vi "rs3 Set All Advanced4.vi"(0 "Set Color Corr":bool=TRUE, 1 "Depth Presets":T2(ring), 2 "Color Presets":T1(ring), 7 "error in (no error)":errorcluster, 8 "device in":u64=370866768, 10 "ST_CensusEnable":cluster{"uDiameter":u32, "vDiameter":u32}={"uDiameter"=9, "vDiameter"=9}, 12 "ST_AE_Control":cluster{"meanIntensitySetpoint":u32}={"meanIntensitySetpoint"=400}, 16 "Depth Table":T3={"depthUnits, um"=1000, "depthClampMin"=0, "depthClampMax"=65535, "disparityMultiplier"=0, "disparityShift"=0}, 17 "ST RAU vector":T9={"minWest"=1, "minEast"=1, "minWEsum"=1, "minNorth"=1, "minSouth"=1, "minNSSum"=1, "uStrink"=1, "vShrink"=1}, 19 "ST Color Control":T8, 20 "depth control":T4={"plusIncrement"=10, "MinusDecrement"=10, "deepSeaMedianThreshold"=528, "scoreThreshA"=10, "scoreThreshB"=1023, "textureDifferenceThreshold"=0, "textureCountThreshold"=0, "deepSeaSecondPeakThreshold"=27, "deepSeaNeighborThreshold"=20, "IrAgreeThreshold"=70}, 21 "STColorCorrection":T11={"colorCorrection 1"=0.54785156, "colorCorrection 2"=0.32910156, "colorCorrection 3"=0.8222656, "colorCorrection 4"=0.109375, "colorCorrection 5"=-0.40527344, "colorCorrection 6"=-1.5253906, "colorCorrection 7"=0.95703125, "colorCorrection 8"=0.89160156, "colorCorrection 9"=0.7675781, "colorCorrection 10"=-0.4794922, "colorCorrection 11"=0.047851562, "colorCorrection 12"=-0.2705078}, 22 "HDAD":T12={"lambdaCensus"=26.0, "lambdaAD"=2100.0, "ignoreSAD"=0}, 23 "ST RSM":T10={"rsmBypass"=0, "diffThresh"=7.0, "sloRauDiffThresh"=3.0, "removeThresh"=33}, 24 "ST SLO Penalty":T5={"sloK1Penalty"=44, "sloK2Penalty"=502, "sloK1PenaltyMod1"=23, "sloK2PenaltyMod1"=237, "sloK1PenaltyMod2"=219, "sloK2PenaltyMod2"=113}, 25 "ST SLO Threshold":T6={"SLOdiffThresholdRed"=300, "SLODiffThresholdGreen"=300, "SLODiffThresholdBlue"=300}, 26 "ST Rau Threshold":T7={"rauDiffThresholdRed"=600, "rauDiffThresholdGreen"=600, "rauDiffThresholdBlue"=600}) -> (14 "Set advanced error":string, 18 "Dev out":u64=370866768, 27 "error out":errorcluster)   [LabVIEW 2017, in "libRealSense3.lvlib"]
doc: "The RealSense D4xx cameras are based on a stereo algorithm that has been accelerated as a fixed-function inside an ASIC. There are many parameters that affect the calculation of the depth. The basic task is to solve the correspondance problem - i.e. figure out which patches in the left image match up to those in the right image by doing a search along an epipolar line (x-axis). The x-axis difference for each object point is known as the disparity. \n\nIn general depth can be estimated for most points in the scene, but some points will have a very low confidence because 1. they are may be occluded (not seen by both imagers), or 2. have very little texture on them which will lead to an ambiquity (ex. when looking at a completely uniform white wall it, there are no best correspondances).\n\nThis VI allows you to set the many parameters that affect the algorith, as well as the color reproduction. \nNote that the color correction matrix will NOT have any effect on the depth calculations."
uses:
  <vilib>/addons/RealSense/libRealSense3.lvlib
panel:
  # "RS3 Set All Advanced 4"
  # "(C) 2017 Intel Corp.,  AGJ"
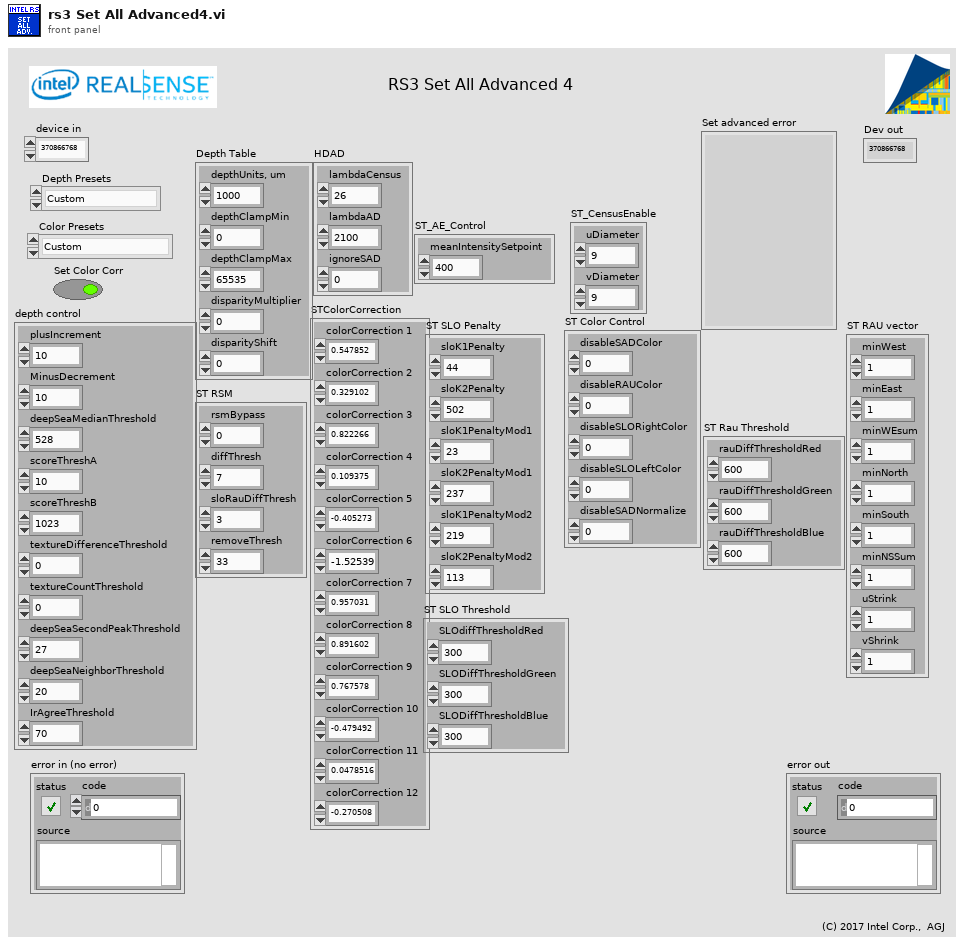
[diagram p1: front panel]
types:
  T1 = enum16{"Custom", "RS400 (DS5p)", "RS400 (DS5p) 2", "RS400 (DS5p) 3", "RS400 (DS5p) 4", "RS400 (DS5p) 5", "RS410 (DS5a)", "RS410 (DS5a) 2", "DS410 (DS5a) 3", "DS410 (DS5a) 4", "DS410+IR", "DS5LR", "DS5LR-2", "DS5LR no pattern", "RS410 Remove IR", "RS410 Remove IR 2", "DS5micro", "D435"}
  T2 = enum16{"Custom", "Original", "New Depth 1", "New Depth 2", "Depth Active 1", "Active 3D Scan", "Active Short A", "Active Short C", "Face", "Face2", "Best Box", "High Density", "Medium Density", "High Accuracy", "Hand", "Short Range", "Flat wall", "Load .JSON", "Load .JSON2"}
  T3 = cluster{"depthUnits, um":u32, "depthClampMin":u32, "depthClampMax":u32, "disparityMultiplier":u32, "disparityShift":u32}
  T4 = cluster{"plusIncrement":u32, "MinusDecrement":u32, "deepSeaMedianThreshold":u32, "scoreThreshA":u32, "scoreThreshB":u32, "textureDifferenceThreshold":u32, "textureCountThreshold":u32, "deepSeaSecondPeakThreshold":u32, "deepSeaNeighborThreshold":u32, "IrAgreeThreshold":u32}
  T5 = cluster{"sloK1Penalty":u32, "sloK2Penalty":u32, "sloK1PenaltyMod1":u32, "sloK2PenaltyMod1":u32, "sloK1PenaltyMod2":u32, "sloK2PenaltyMod2":u32}
  T6 = cluster{"SLOdiffThresholdRed":u32, "SLODiffThresholdGreen":u32, "SLODiffThresholdBlue":u32}
  T7 = cluster{"rauDiffThresholdRed":u32, "rauDiffThresholdGreen":u32, "rauDiffThresholdBlue":u32}
  T8 = cluster{"disableSADColor":u32, "disableRAUColor":u32, "disableSLORightColor":u32, "disableSLOLeftColor":u32, "disableSADNormalize":u32}
  T9 = cluster{"minWest":u32, "minEast":u32, "minWEsum":u32, "minNorth":u32, "minSouth":u32, "minNSSum":u32, "uStrink":u32, "vShrink":u32}
  T10 = cluster{"rsmBypass":u32, "diffThresh":sgl, "sloRauDiffThresh":sgl, "removeThresh":u32}
  T11 = cluster{"colorCorrection 1":sgl, "colorCorrection 2":sgl, "colorCorrection 3":sgl, "colorCorrection 4":sgl, "colorCorrection 5":sgl, "colorCorrection 6":sgl, "colorCorrection 7":sgl, "colorCorrection 8":sgl, "colorCorrection 9":sgl, "colorCorrection 10":sgl, "colorCorrection 11":sgl, "colorCorrection 12":sgl}
  T12 = cluster{"lambdaCensus":sgl, "lambdaAD":sgl, "ignoreSAD":u32}
  T13 = cluster{"rsmBypass (56)":u32, "diffThresh (57)":sgl, "sloRauDiffThresh(58)":sgl, "removeThresh(59)":u32}
  T14 = cluster{"depth control":cluster{"plusIncrement":u32, "MinusDecrement":u32, "deepSeaMedianThreshold":u32, "scoreThreshA":u32, "scoreThreshB":u32, "textureDifferenceThreshold":u32, "textureCountThreshold":u32, "deepSeaSecondPeakThreshold":u32, "deepSeaNeighborThreshold":u32, "IrAgreeThreshold":u32}, "STColorCorrection output":cluster{"colorCorrection 1":sgl, "colorCorrection 2":sgl, "colorCorrection 3":sgl, "colorCorrection 4":sgl, "colorCorrection 5":sgl, "colorCorrection 6":sgl, "colorCorrection 7":sgl, "colorCorrection 8":sgl, "colorCorrection 9":sgl, "colorCorrection 10":sgl, "colorCorrection 11":sgl, "colorCorrection 12":sgl}, "HDAD":cluster{"lambdaCensus":sgl, "lambdaAD":sgl, "ignoreSAD":u32}, "ST RSM":cluster{"rsmBypass":u32, "diffThresh":sgl, "sloRauDiffThresh":sgl, "removeThresh":u32}, "ST SLO Penalty":cluster{"sloK1Penalty":u32, "sloK2Penalty":u32, "sloK1PenaltyMod1":u32, "sloK2PenaltyMod1":u32, "sloK1PenaltyMod2":u32, "sloK2PenaltyMod2":u32}, "ST SLO Threshold":cluster{"SLOdiffThresholdRed":u32, "SLODiffThresholdGreen":u32, "SLODiffThresholdBlue":u32}, "ST Rau Threshold":cluster{"rauDiffThresholdRed":u32, "rauDiffThresholdGreen":u32, "rauDiffThresholdBlue":u32}, "ST Color Control":cluster{"disableSADColor":u32, "disableRAUColor":u32, "disableSLORightColor":u32, "disableSLOLeftColor":u32, "disableSADNormalize":u32}, "ST RAU vector":cluster{"minWest":u32, "minEast":u32, "minWEsum":u32, "minNorth":u32, "minSouth":u32, "minNSSum":u32, "uStrink":u32, "vShrink":u32}, "Depth Table":cluster{"depthUnits, um":u32, "depthClampMin":u32, "depthClampMax":u32, "disparityMultiplier":u32, "disparityShift":u32}, "ST_AE_Control":cluster{"meanIntensitySetpoint":u32}, "ST_CensusEnable":cluster{"uDiameter":u32, "vDiameter":u32}}
  T15 = cluster{"depthUnits, um":u32, "depthClampMin":u32, "depthClampMax":u32, "disparityMultiplier":u32, "disparityShift(0-127)":u32}
  T16 = cluster{"minWest (60)":u32, "minEast (61)":u32, "minWEsum (62)":u32, "minNorth (63)":u32, "minSouth (64)":u32, "minNSSum(65)":u32, "uStrink (66)":u32, "vShrink (67)":u32}
  T17 = cluster{"rauDiffThreshRed(73)":u32, "rauDiffThreshGreen(74)":u32, "rauDiffThreshBlue(75)":u32}
  T18 = cluster{"sloK1Penalty (79)":u32, "sloK2Penalty (80)":u32, "sloK1PenaltyMod1(81)":u32, "sloK2PenaltyMod1(82)":u32, "sloK1PenaltyMod2(83)":u32, "sloK2PenaltyMod2(84)":u32}
  T19 = cluster{"SLOdiffThreshRed(76)":u32, "SLODiffThreshGreen(77)":u32, "SLODiffThreshBlue(78)":u32}
  T20 = cluster{"disableSADColor(68)":u32, "disableRAUColor(69)":u32, "disableSLORightColor(70)":u32, "disableSLOLeftColor(71)":u32, "disableSADNormalize(72)":u32}
  T21 = cluster{"plusIncrement (47)":u32, "MinusDecrement (46)":u32, "deepSeaMedianThreshold (48)":u32, "scoreThreshA(49)":u32, "scoreThreshB (50)":u32, "textureDifferenceThreshold (52)":u32, "textureCountThreshold (51)":u32, "deepSea2ndPeakThresh.(53)":u32, "deepSeaNeighborThresh.(54)":u32, "LRAgreeThreshold (55)":u32}
  T22 = cluster{"plusIncrement (47)":u32, "MinusDecrement (46)":u32, "deepSeaMedianThreshold (48)":u32, "scoreThreshA(49)":u32, "scoreThreshB (50)":u32, "textureDifferenceThreshold (52)":u32, "textureCountThreshold (51)":u32, "deepSea2ndPeakThresh.(53)":u32, "deepSeaNeighborThresh.(54)":u32, "IrAgreeThreshold (55)":u32}
  T23 = cluster{"DS5p- 1":sgl, "colorCorrection 2":sgl, "colorCorrection 3":sgl, "colorCorrection 4":sgl, "colorCorrection 5":sgl, "colorCorrection 6":sgl, "colorCorrection 7":sgl, "colorCorrection 8":sgl, "colorCorrection 9":sgl, "colorCorrection 10":sgl, "colorCorrection 11":sgl, "colorCorrection 12":sgl}
  T24 = cluster{"Color 0":dbl, "Color 1":dbl, "Color 2":dbl, "Color 3":dbl, "Color 4":dbl, "Color 5":dbl, "Color 6":dbl, "Color 7":dbl, "Color 8":dbl, "Color 9":dbl, "Color 10":dbl, "Color 11":dbl}
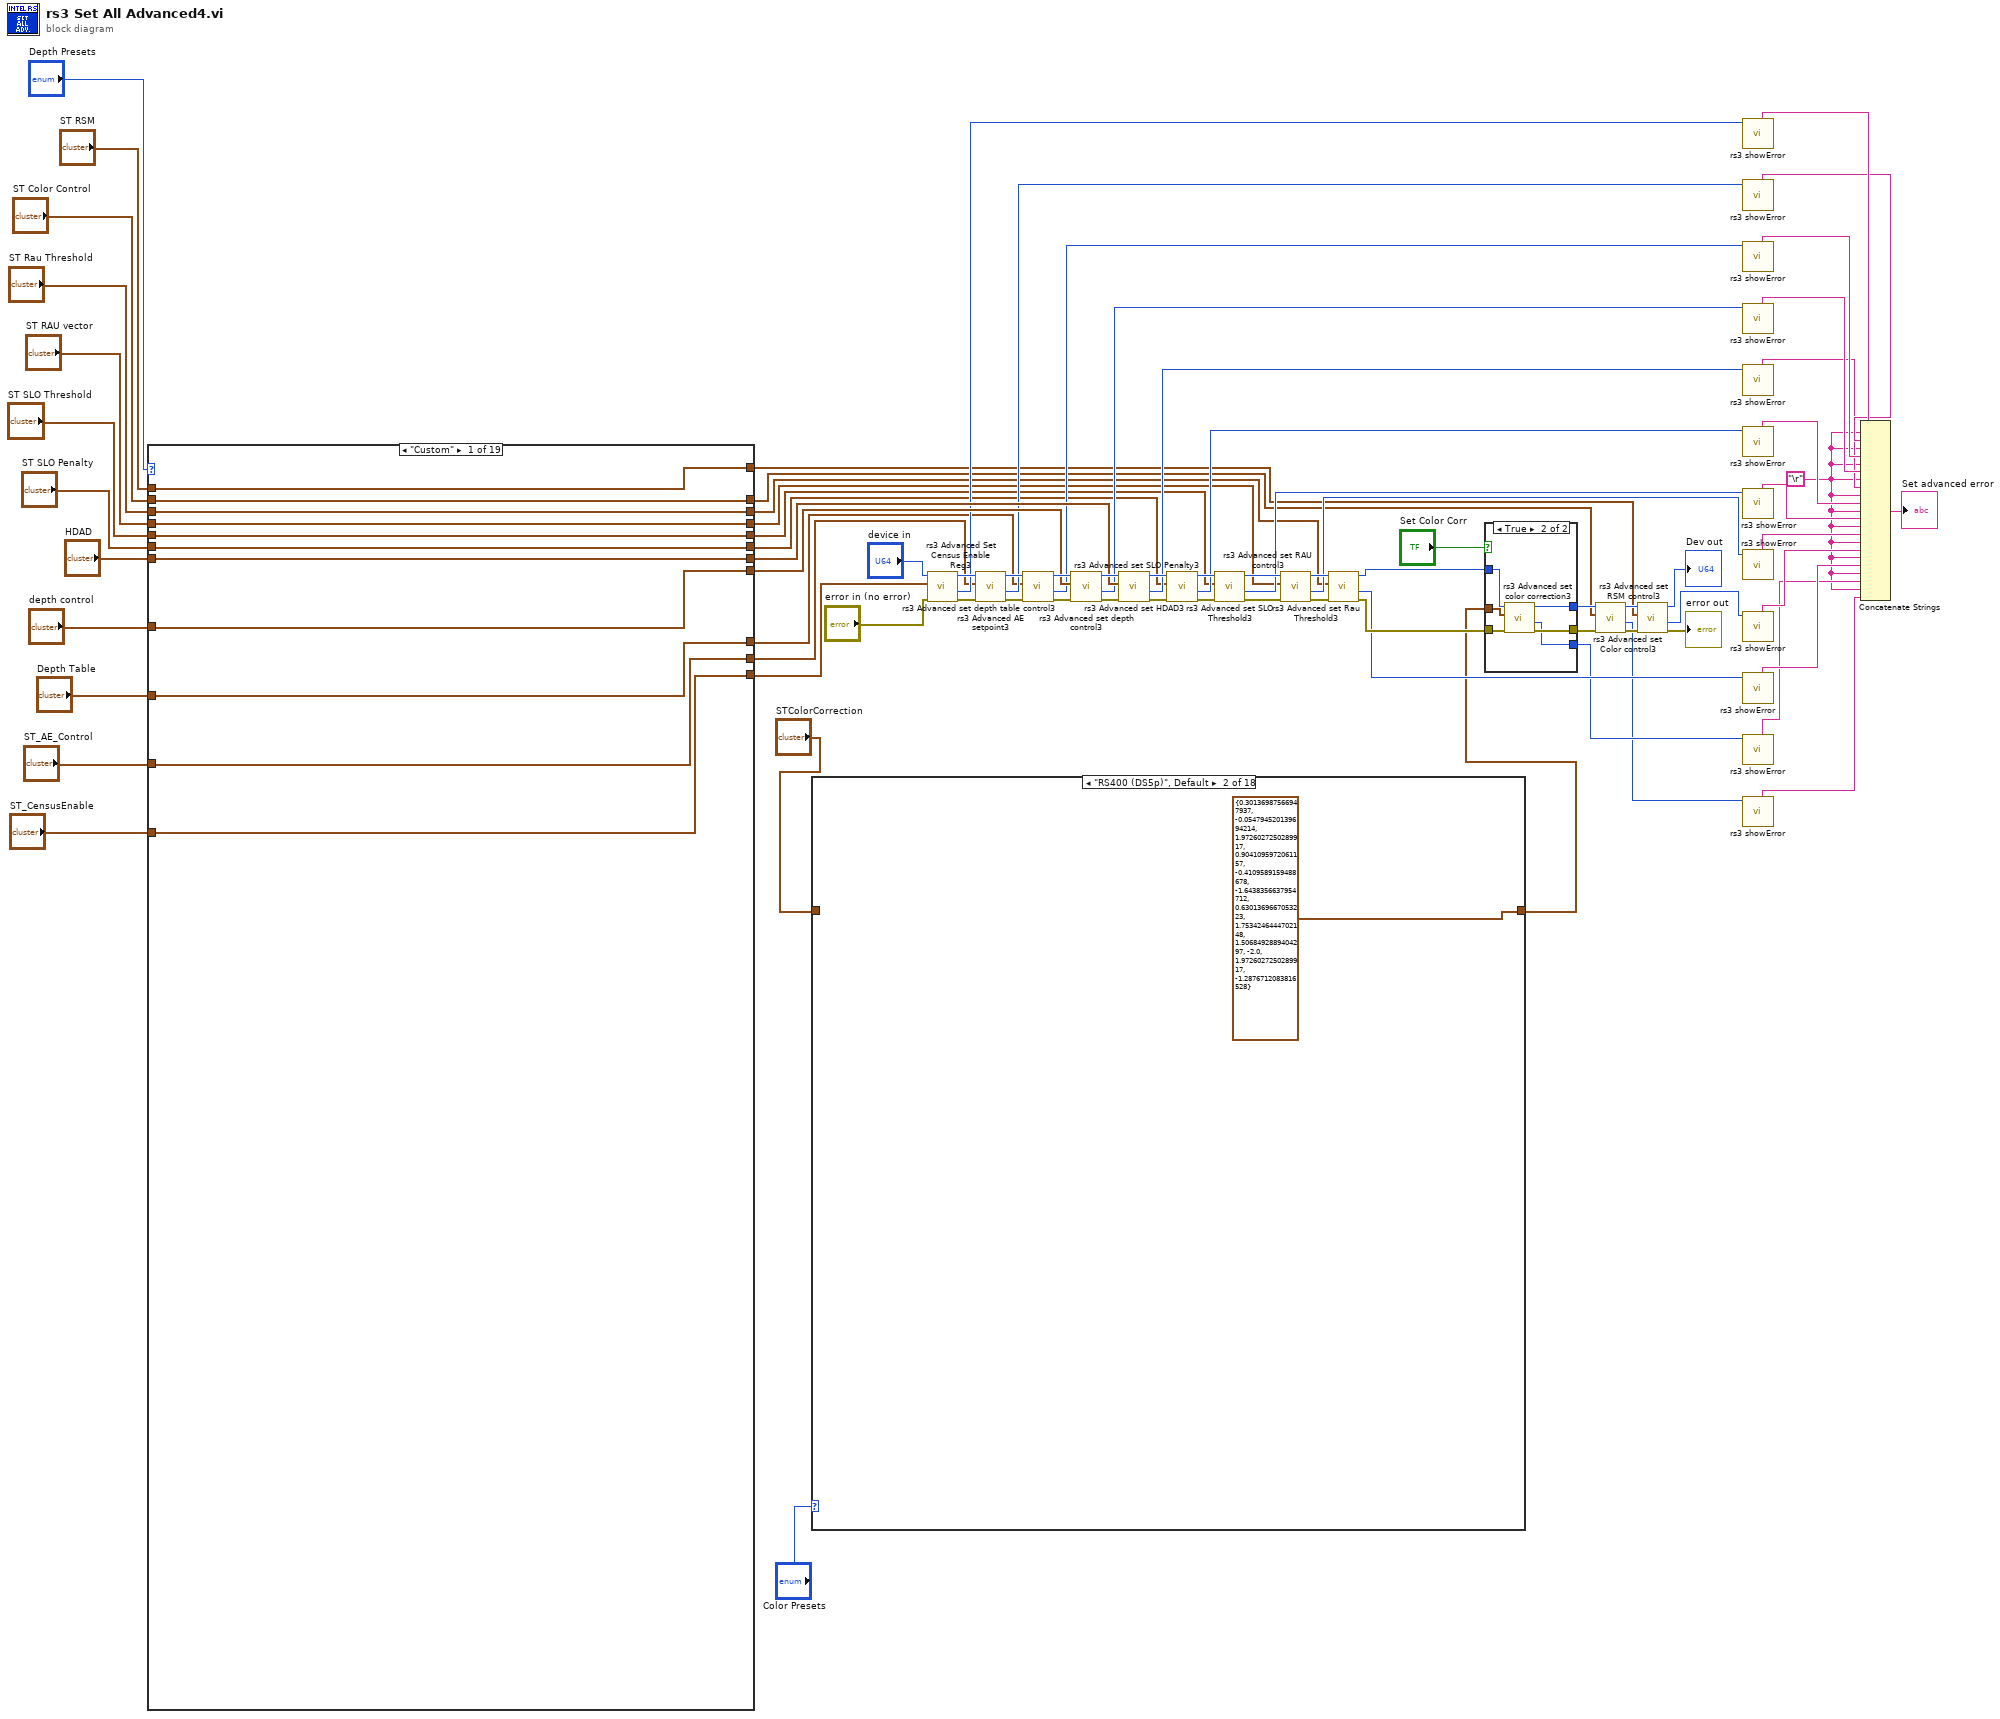
[diagram p0: block diagram]
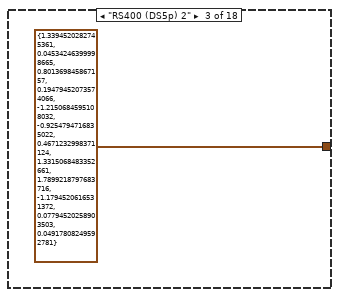
[diagram p3: hidden frame]
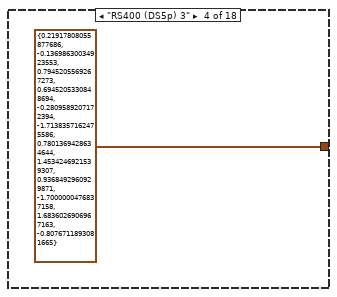
[diagram p4: hidden frame]
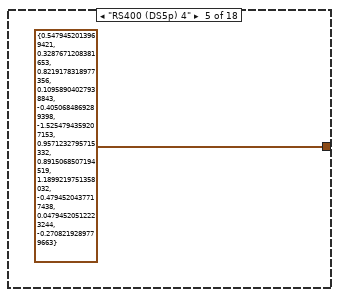
[diagram p5: hidden frame]
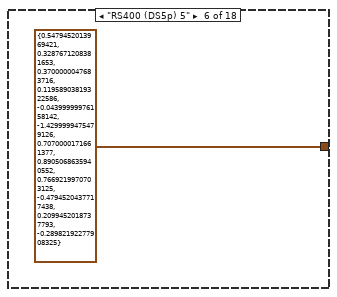
[diagram p6: hidden frame]
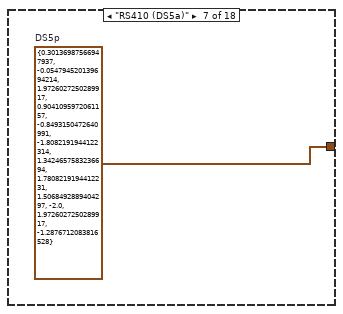
[diagram p7: hidden frame]
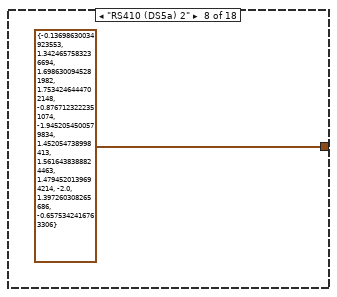
[diagram p8: hidden frame]
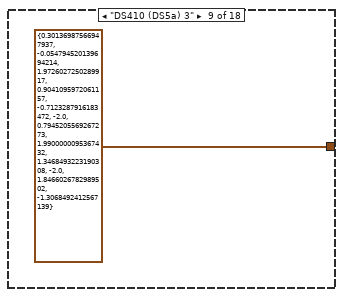
[diagram p9: hidden frame]
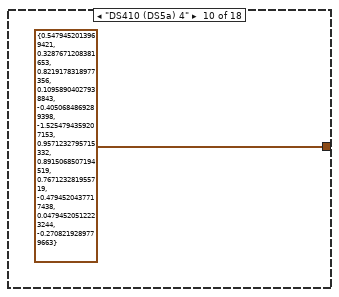
[diagram p10: hidden frame]
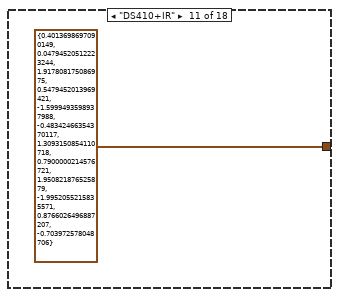
[diagram p11: hidden frame]
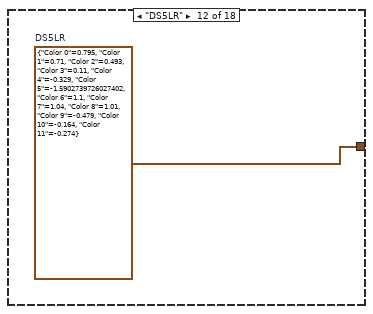
[diagram p12: hidden frame]
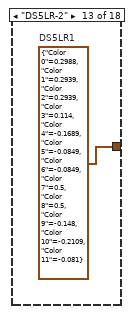
[diagram p13: hidden frame]
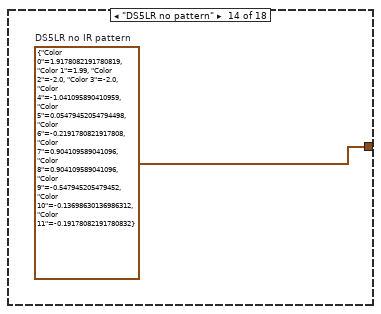
[diagram p14: hidden frame]
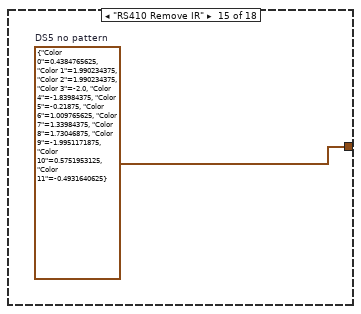
[diagram p15: hidden frame]
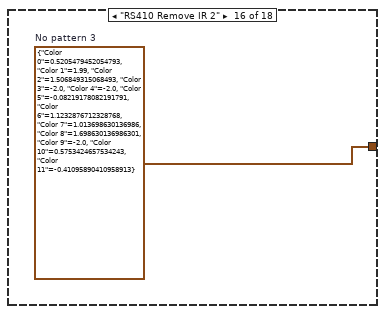
[diagram p16: hidden frame]
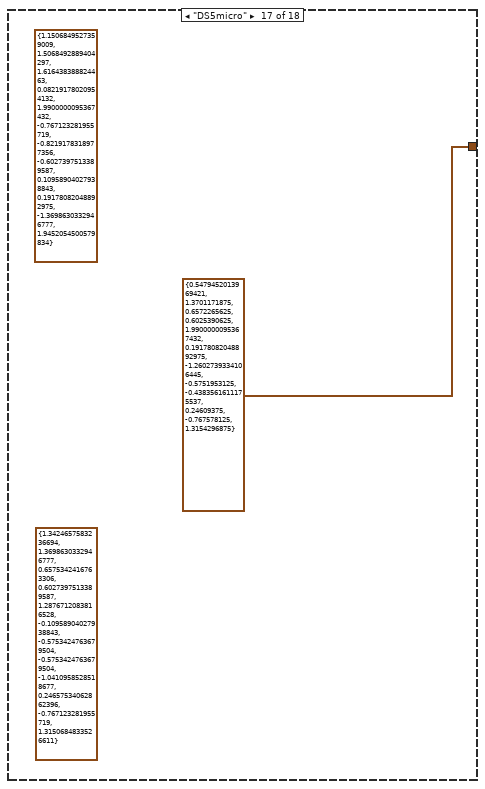
[diagram p17: hidden frame]
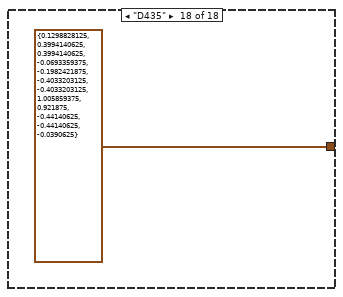
[diagram p18: hidden frame]
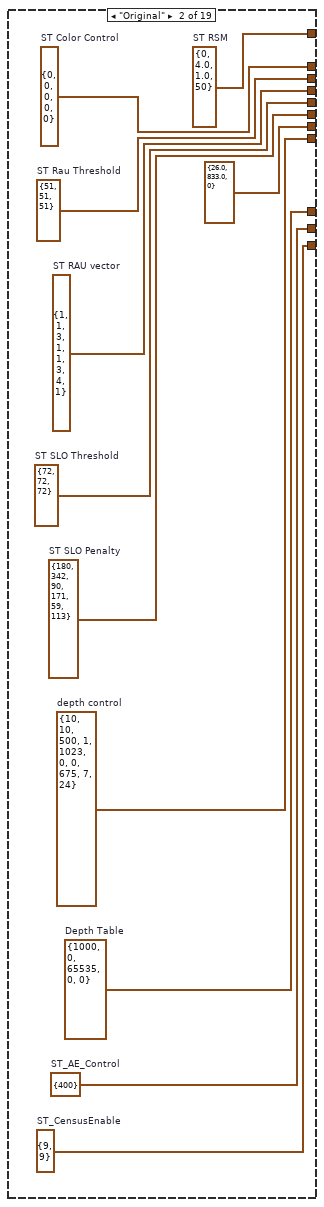
[diagram p19: hidden frame]
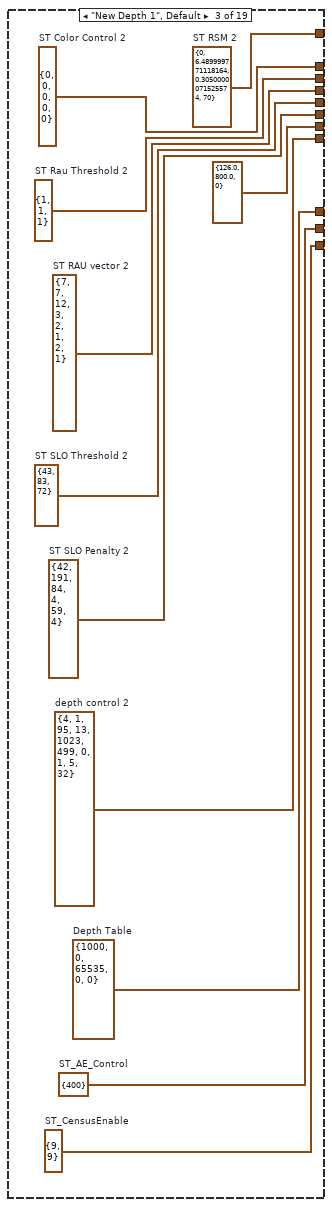
[diagram p20: hidden frame]
diagram:
  w23 = "\r"
  n1 = case shown="\"Custom\"" "Depth Presets" {
    tunnel: [w90 w100 w112 w123 w134 w138 w149 w160 w176 w186 w197 w204 w217 w229 w241 w253 w265 w280 w294] -> w50
    tunnel: [w84 w99 w111 w122 w133 T13 {"rsmBypass (56)"=0, "diffThresh (57)"=1.0367311, "sloRauDiffThresh(58)"=151.0, "removeThresh(59)"=1} ("ST RSM 2") w156 w167 w178 w183 w194 w209 w222 w234 w246 w258 w270 w282 w296] -> w12
    tunnel: [w85 w94 w110 w121 w132 w145 w155 w166 w177 w184 w195 w211 w224 w236 w248 w260 w272 w279 w293] -> w14
    tunnel: [w86 w95 w109 w120 w131 w144 w154 w165 w174 w185 w196 w207 w220 w232 w244 w256 w268 w283 w297] -> w15
    tunnel: [w83 w98 w108 w119 w130 w143 w153 w164 w173 w187 w198 w203 w216 w228 w240 w252 w264 w286 w300] -> w10
    tunnel: [w87 w97 w107 w118 w129 w142 w152 w163 w171 w188 w199 w202 w215 w227 w239 w251 w263 w285 w299] -> w17
    tunnel: [w88 w96 w106 w117 w128 w141 w151 w162 w175 w189 w200 w201 w214 w226 w238 w250 w262 w284 w298] -> w20
    tunnel: [w89 T12 {"lambdaCensus"=26.0, "lambdaAD"=833.0, "ignoreSAD"=0} ("HDAD 2") T12 {"lambdaCensus"=126.0, "lambdaAD"=800.0, "ignoreSAD"=0} ("HDAD 2") T12 {"lambdaCensus"=200.0, "lambdaAD"=1900.0, "ignoreSAD"=0} ("HDAD 2") T12 {"lambdaCensus"=216.0, "lambdaAD"=1400.0, "ignoreSAD"=0} ("HDAD 2") T12 {"lambdaCensus"=26.0, "lambdaAD"=833.0, "ignoreSAD"=0} ("HDAD 2") T12 {"lambdaCensus"=100.0, "lambdaAD"=1600.0, "ignoreSAD"=0} ("HDAD 2") w161 w172 T12 {"lambdaCensus"=26.0, "lambdaAD"=2100.0, "ignoreSAD"=0} ("HDAD*") T12 {"lambdaCensus"=15.0, "lambdaAD"=618.0, "ignoreSAD"=0} ("HDAD*") w210 w223 w235 w247 w259 w271 w281 w295] -> w48
    tunnel: [w81 w91 w102 w113 w124 w135 w146 w158 w168 w179 w190 w205 w218 w230 w242 w254 w266 w273 w289] -> w6
    tunnel: [w82 w92 w103 w114 w125 w136 w147 w157 w169 w180 w191 w206 w219 w231 w243 w255 w267 w274 w288] -> w8
    tunnel: [w80 w93 w104 w115 w126 w137 w148 w159 w170 w181 w192 w208 w221 w233 w245 w257 w269 w275 w287] -> w4
    tunnel: "depth control" -> [w90 _ _ _ _ _ _ _ _ _ _ _ _ _ _ _ _ _ _]
    tunnel: "HDAD" -> [w89 _ _ _ _ _ _ _ _ _ _ _ _ _ _ _ _ _ _]
    tunnel: "ST SLO Penalty" -> [w88 _ _ _ _ _ _ _ _ _ _ _ _ _ _ _ _ _ _]
    tunnel: "ST SLO Threshold" -> [w87 _ _ _ _ _ _ _ _ _ _ _ _ _ _ _ _ _ _]
    tunnel: "ST RAU vector" -> [w85 _ _ _ _ _ _ _ _ _ _ _ _ _ _ _ _ _ _]
    tunnel: "ST Rau Threshold" -> [w86 _ _ _ _ _ _ _ _ _ _ _ _ _ _ _ _ _ _]
    tunnel: "ST RSM" -> [w84 _ _ _ _ _ _ _ _ _ _ _ _ _ _ _ _ _ _]
    tunnel: "ST Color Control" -> [w83 _ _ _ _ _ _ _ _ _ _ _ _ _ _ _ _ _ _]
    tunnel: "ST_CensusEnable" -> [w82 _ _ _ _ _ _ _ _ _ _ _ _ _ _ _ _ _ _]
    tunnel: "ST_AE_Control" -> [w81 _ _ _ _ _ _ _ _ _ _ _ _ _ _ _ _ _ _]
    tunnel: "Depth Table" -> [w80 _ _ _ _ _ _ _ _ _ _ _ _ _ _ _ _ _ _]
    frame "Custom" {
    }
    frame "Original" {
      w92 = cluster{"uDiameter":u32, "vDiameter":u32} {"uDiameter"=9, "vDiameter"=9}  # ST_CensusEnable
      w93 = T15 {"depthUnits, um"=1000, "depthClampMin"=0, "depthClampMax"=65535, "disparityMultiplier"=0, "disparityShift(0-127)"=0}  # Depth Table
      w91 = cluster{"meanIntensitySetpoint":u32} {"meanIntensitySetpoint"=400}  # ST_AE_Control
      w94 = T16 {"minWest (60)"=1, "minEast (61)"=1, "minWEsum (62)"=3, "minNorth (63)"=1, "minSouth (64)"=1, "minNSSum(65)"=3, "uStrink (66)"=4, "vShrink (67)"=1}  # ST RAU vector
      w95 = T17 {"rauDiffThreshRed(73)"=51, "rauDiffThreshGreen(74)"=51, "rauDiffThreshBlue(75)"=51}  # ST Rau Threshold
      w96 = T18 {"sloK1Penalty (79)"=180, "sloK2Penalty (80)"=342, "sloK1PenaltyMod1(81)"=90, "sloK2PenaltyMod1(82)"=171, "sloK1PenaltyMod2(83)"=59, "sloK2PenaltyMod2(84)"=113}  # ST SLO Penalty
      w97 = T19 {"SLOdiffThreshRed(76)"=72, "SLODiffThreshGreen(77)"=72, "SLODiffThreshBlue(78)"=72}  # ST SLO Threshold
      w98 = T20 {"disableSADColor(68)"=0, "disableRAUColor(69)"=0, "disableSLORightColor(70)"=0, "disableSLOLeftColor(71)"=0, "disableSADNormalize(72)"=0}  # ST Color Control
      w99 = T13 {"rsmBypass (56)"=0, "diffThresh (57)"=4.0, "sloRauDiffThresh(58)"=1.0, "removeThresh(59)"=50}  # ST RSM
      w100 = T21 {"plusIncrement (47)"=10, "MinusDecrement (46)"=10, "deepSeaMedianThreshold (48)"=500, "scoreThreshA(49)"=1, "scoreThreshB (50)"=1023, "textureDifferenceThreshold (52)"=0, "textureCountThreshold (51)"=0, "deepSea2ndPeakThresh.(53)"=675, "deepSeaNeighborThresh.(54)"=7, "LRAgreeThreshold (55)"=24}  # depth control
    }
    frame "New Depth 1", Default {
      w103 = cluster{"uDiameter":u32, "vDiameter":u32} {"uDiameter"=9, "vDiameter"=9}  # ST_CensusEnable
      w104 = T15 {"depthUnits, um"=1000, "depthClampMin"=0, "depthClampMax"=65535, "disparityMultiplier"=0, "disparityShift(0-127)"=0}  # Depth Table
      w102 = cluster{"meanIntensitySetpoint":u32} {"meanIntensitySetpoint"=400}  # ST_AE_Control
      w106 = T18 {"sloK1Penalty (79)"=42, "sloK2Penalty (80)"=191, "sloK1PenaltyMod1(81)"=84, "sloK2PenaltyMod1(82)"=4, "sloK1PenaltyMod2(83)"=59, "sloK2PenaltyMod2(84)"=4}  # ST SLO Penalty 2
      w107 = T19 {"SLOdiffThreshRed(76)"=43, "SLODiffThreshGreen(77)"=83, "SLODiffThreshBlue(78)"=72}  # ST SLO Threshold 2
      w108 = T20 {"disableSADColor(68)"=0, "disableRAUColor(69)"=0, "disableSLORightColor(70)"=0, "disableSLOLeftColor(71)"=0, "disableSADNormalize(72)"=0}  # ST Color Control 2
      w109 = T17 {"rauDiffThreshRed(73)"=1, "rauDiffThreshGreen(74)"=1, "rauDiffThreshBlue(75)"=1}  # ST Rau Threshold 2
      w110 = T16 {"minWest (60)"=7, "minEast (61)"=7, "minWEsum (62)"=12, "minNorth (63)"=3, "minSouth (64)"=2, "minNSSum(65)"=1, "uStrink (66)"=2, "vShrink (67)"=1}  # ST RAU vector 2
      w111 = T13 {"rsmBypass (56)"=0, "diffThresh (57)"=6.49, "sloRauDiffThresh(58)"=0.305, "removeThresh(59)"=70}  # ST RSM 2
      w112 = T22 {"plusIncrement (47)"=4, "MinusDecrement (46)"=1, "deepSeaMedianThreshold (48)"=95, "scoreThreshA(49)"=13, "scoreThreshB (50)"=1023, "textureDifferenceThreshold (52)"=499, "textureCountThreshold (51)"=0, "deepSea2ndPeakThresh.(53)"=1, "deepSeaNeighborThresh.(54)"=5, "IrAgreeThreshold (55)"=32}  # depth control 2
    }
    frame "New Depth 2" {
      w114 = cluster{"uDiameter":u32, "vDiameter":u32} {"uDiameter"=9, "vDiameter"=9}  # ST_CensusEnable
      w115 = T15 {"depthUnits, um"=1000, "depthClampMin"=0, "depthClampMax"=65535, "disparityMultiplier"=0, "disparityShift(0-127)"=0}  # Depth Table
      w113 = cluster{"meanIntensitySetpoint":u32} {"meanIntensitySetpoint"=400}  # ST_AE_Control
      w117 = T18 {"sloK1Penalty (79)"=42, "sloK2Penalty (80)"=191, "sloK1PenaltyMod1(81)"=84, "sloK2PenaltyMod1(82)"=4, "sloK1PenaltyMod2(83)"=59, "sloK2PenaltyMod2(84)"=4}  # ST SLO Penalty 2
      w118 = T19 {"SLOdiffThreshRed(76)"=100, "SLODiffThreshGreen(77)"=100, "SLODiffThreshBlue(78)"=100}  # ST SLO Threshold 2
      w119 = T20 {"disableSADColor(68)"=0, "disableRAUColor(69)"=0, "disableSLORightColor(70)"=0, "disableSLOLeftColor(71)"=0, "disableSADNormalize(72)"=0}  # ST Color Control 2
      w120 = T17 {"rauDiffThreshRed(73)"=50, "rauDiffThreshGreen(74)"=50, "rauDiffThreshBlue(75)"=50}  # ST Rau Threshold 2
      w121 = T16 {"minWest (60)"=1, "minEast (61)"=1, "minWEsum (62)"=9, "minNorth (63)"=3, "minSouth (64)"=2, "minNSSum(65)"=1, "uStrink (66)"=2, "vShrink (67)"=1}  # ST RAU vector 2
      w122 = T13 {"rsmBypass (56)"=0, "diffThresh (57)"=6.49, "sloRauDiffThresh(58)"=0.305, "removeThresh(59)"=50}  # ST RSM 2
      w123 = T22 {"plusIncrement (47)"=4, "MinusDecrement (46)"=1, "deepSeaMedianThreshold (48)"=95, "scoreThreshA(49)"=13, "scoreThreshB (50)"=1023, "textureDifferenceThreshold (52)"=499, "textureCountThreshold (51)"=0, "deepSea2ndPeakThresh.(53)"=1, "deepSeaNeighborThresh.(54)"=5, "IrAgreeThreshold (55)"=200}  # depth control 2
    }
    frame "Depth Active 1" {
      w125 = cluster{"uDiameter":u32, "vDiameter":u32} {"uDiameter"=9, "vDiameter"=9}  # ST_CensusEnable
      w126 = T15 {"depthUnits, um"=1000, "depthClampMin"=0, "depthClampMax"=65535, "disparityMultiplier"=0, "disparityShift(0-127)"=0}  # Depth Table
      w124 = cluster{"meanIntensitySetpoint":u32} {"meanIntensitySetpoint"=400}  # ST_AE_Control
      w128 = T18 {"sloK1Penalty (79)"=10, "sloK2Penalty (80)"=60, "sloK1PenaltyMod1(81)"=84, "sloK2PenaltyMod1(82)"=56, "sloK1PenaltyMod2(83)"=59, "sloK2PenaltyMod2(84)"=4}  # ST SLO Penalty 2
      w129 = T19 {"SLOdiffThreshRed(76)"=200, "SLODiffThreshGreen(77)"=200, "SLODiffThreshBlue(78)"=200}  # ST SLO Threshold 2
      w130 = T20 {"disableSADColor(68)"=0, "disableRAUColor(69)"=0, "disableSLORightColor(70)"=0, "disableSLOLeftColor(71)"=0, "disableSADNormalize(72)"=0}  # ST Color Control 2
      w131 = T17 {"rauDiffThreshRed(73)"=70, "rauDiffThreshGreen(74)"=70, "rauDiffThreshBlue(75)"=70}  # ST Rau Threshold 2
      w132 = T16 {"minWest (60)"=7, "minEast (61)"=7, "minWEsum (62)"=12, "minNorth (63)"=3, "minSouth (64)"=2, "minNSSum(65)"=1, "uStrink (66)"=2, "vShrink (67)"=1}  # ST RAU vector 2
      w133 = T13 {"rsmBypass (56)"=0, "diffThresh (57)"=6.49, "sloRauDiffThresh(58)"=0.305, "removeThresh(59)"=60}  # ST RSM 2
      w134 = T22 {"plusIncrement (47)"=4, "MinusDecrement (46)"=1, "deepSeaMedianThreshold (48)"=95, "scoreThreshA(49)"=13, "scoreThreshB (50)"=1023, "textureDifferenceThreshold (52)"=499, "textureCountThreshold (51)"=0, "deepSea2ndPeakThresh.(53)"=1, "deepSeaNeighborThresh.(54)"=5, "IrAgreeThreshold (55)"=82}  # depth control 2
    }
    frame "Active 3D Scan" {
      w136 = cluster{"uDiameter":u32, "vDiameter":u32} {"uDiameter"=9, "vDiameter"=9}  # ST_CensusEnable
      w137 = T15 {"depthUnits, um"=1000, "depthClampMin"=0, "depthClampMax"=65535, "disparityMultiplier"=0, "disparityShift(0-127)"=0}  # Depth Table
      w135 = cluster{"meanIntensitySetpoint":u32} {"meanIntensitySetpoint"=400}  # ST_AE_Control
      w138 = T22 {"plusIncrement (47)"=19, "MinusDecrement (46)"=4, "deepSeaMedianThreshold (48)"=554, "scoreThreshA(49)"=1, "scoreThreshB (50)"=632, "textureDifferenceThreshold (52)"=0, "textureCountThreshold (51)"=31, "deepSea2ndPeakThresh.(53)"=665, "deepSeaNeighborThresh.(54)"=126, "IrAgreeThreshold (55)"=11}  # depth control 2
      w141 = T18 {"sloK1Penalty (79)"=93, "sloK2Penalty (80)"=473, "sloK1PenaltyMod1(81)"=70, "sloK2PenaltyMod1(82)"=123, "sloK1PenaltyMod2(83)"=92, "sloK2PenaltyMod2(84)"=409}  # ST SLO Penalty 2
      w142 = T19 {"SLOdiffThreshRed(76)"=46, "SLODiffThreshGreen(77)"=442, "SLODiffThreshBlue(78)"=105}  # ST SLO Threshold 2
      w143 = T20 {"disableSADColor(68)"=0, "disableRAUColor(69)"=0, "disableSLORightColor(70)"=0, "disableSLOLeftColor(71)"=0, "disableSADNormalize(72)"=0}  # ST Color Control 2
      w144 = T17 {"rauDiffThreshRed(73)"=46, "rauDiffThreshGreen(74)"=442, "rauDiffThreshBlue(75)"=105}  # ST Rau Threshold 2
      w145 = T16 {"minWest (60)"=5, "minEast (61)"=7, "minWEsum (62)"=12, "minNorth (63)"=1, "minSouth (64)"=3, "minNSSum(65)"=7, "uStrink (66)"=4, "vShrink (67)"=1}  # ST RAU vector 2
    }
    frame "Active Short A" {
      w147 = cluster{"uDiameter":u32, "vDiameter":u32} {"uDiameter"=3, "vDiameter"=3}  # ST_CensusEnable
      w148 = T15 {"depthUnits, um"=200, "depthClampMin"=0, "depthClampMax"=65535, "disparityMultiplier"=0, "disparityShift(0-127)"=0}  # Depth Table
      w146 = cluster{"meanIntensitySetpoint":u32} {"meanIntensitySetpoint"=400}  # ST_AE_Control
      w149 = T22 {"plusIncrement (47)"=7, "MinusDecrement (46)"=1, "deepSeaMedianThreshold (48)"=140, "scoreThreshA(49)"=10, "scoreThreshB (50)"=1023, "textureDifferenceThreshold (52)"=499, "textureCountThreshold (51)"=0, "deepSea2ndPeakThresh.(53)"=1, "deepSeaNeighborThresh.(54)"=5, "IrAgreeThreshold (55)"=80}  # depth control 2
      w151 = T18 {"sloK1Penalty (79)"=5, "sloK2Penalty (80)"=30, "sloK1PenaltyMod1(81)"=11, "sloK2PenaltyMod1(82)"=50, "sloK1PenaltyMod2(83)"=56, "sloK2PenaltyMod2(84)"=15}  # ST SLO Penalty 2
      w152 = T19 {"SLOdiffThreshRed(76)"=200, "SLODiffThreshGreen(77)"=200, "SLODiffThreshBlue(78)"=200}  # ST SLO Threshold 2
      w153 = T20 {"disableSADColor(68)"=0, "disableRAUColor(69)"=0, "disableSLORightColor(70)"=0, "disableSLOLeftColor(71)"=0, "disableSADNormalize(72)"=0}  # ST Color Control 2
      w154 = T17 {"rauDiffThreshRed(73)"=200, "rauDiffThreshGreen(74)"=200, "rauDiffThreshBlue(75)"=200}  # ST Rau Threshold 2
      w155 = T16 {"minWest (60)"=3, "minEast (61)"=3, "minWEsum (62)"=13, "minNorth (63)"=1, "minSouth (64)"=1, "minNSSum(65)"=1, "uStrink (66)"=4, "vShrink (67)"=4}  # ST RAU vector 2
      w156 = T13 {"rsmBypass (56)"=0, "diffThresh (57)"=7.5, "sloRauDiffThresh(58)"=0.9, "removeThresh(59)"=72}  # ST RSM 2
    }
    frame "Active Short C" {
      w157 = cluster{"uDiameter":u32, "vDiameter":u32} {"uDiameter"=3, "vDiameter"=3}  # ST_CensusEnable
      w159 = T15 {"depthUnits, um"=200, "depthClampMin"=0, "depthClampMax"=65535, "disparityMultiplier"=0, "disparityShift(0-127)"=0}  # Depth Table
      w158 = cluster{"meanIntensitySetpoint":u32} {"meanIntensitySetpoint"=400}  # ST_AE_Control
      w160 = T22 {"plusIncrement (47)"=10, "MinusDecrement (46)"=10, "deepSeaMedianThreshold (48)"=415, "scoreThreshA(49)"=1, "scoreThreshB (50)"=1023, "textureDifferenceThreshold (52)"=0, "textureCountThreshold (51)"=14, "deepSea2ndPeakThresh.(53)"=56, "deepSeaNeighborThresh.(54)"=108, "IrAgreeThreshold (55)"=8}  # depth control 2
      w161 = T12 {"lambdaCensus"=26.0, "lambdaAD"=958.0, "ignoreSAD"=0}  # HDAD 2
      w162 = T18 {"sloK1Penalty (79)"=203, "sloK2Penalty (80)"=342, "sloK1PenaltyMod1(81)"=109, "sloK2PenaltyMod1(82)"=502, "sloK1PenaltyMod2(83)"=209, "sloK2PenaltyMod2(84)"=14}  # ST SLO Penalty 2
      w163 = T19 {"SLOdiffThreshRed(76)"=889, "SLODiffThreshGreen(77)"=69, "SLODiffThreshBlue(78)"=189}  # ST SLO Threshold 2
      w164 = T20 {"disableSADColor(68)"=0, "disableRAUColor(69)"=0, "disableSLORightColor(70)"=0, "disableSLOLeftColor(71)"=0, "disableSADNormalize(72)"=0}  # ST Color Control 2
      w165 = T17 {"rauDiffThreshRed(73)"=298, "rauDiffThreshGreen(74)"=95, "rauDiffThreshBlue(75)"=675}  # ST Rau Threshold 2
      w166 = T16 {"minWest (60)"=1, "minEast (61)"=1, "minWEsum (62)"=3, "minNorth (63)"=1, "minSouth (64)"=1, "minNSSum(65)"=3, "uStrink (66)"=3, "vShrink (67)"=1}  # ST RAU vector 2
      w167 = T13 {"rsmBypass (56)"=0, "diffThresh (57)"=5.386, "sloRauDiffThresh(58)"=0.9687, "removeThresh(59)"=88}  # ST RSM 2
    }
    frame "Face" {
      w169 = cluster{"uDiameter":u32, "vDiameter":u32} {"uDiameter"=9, "vDiameter"=9}  # ST_CensusEnable
      w170 = T15 {"depthUnits, um"=1000, "depthClampMin"=0, "depthClampMax"=65535, "disparityMultiplier"=0, "disparityShift(0-127)"=0}  # Depth Table
      w168 = cluster{"meanIntensitySetpoint":u32} {"meanIntensitySetpoint"=800}  # ST_AE_Control
      w172 = T12 {"lambdaCensus"=26.0, "lambdaAD"=2100.0, "ignoreSAD"=0}  # HDAD*
      w171 = T19 {"SLOdiffThreshRed(76)"=300, "SLODiffThreshGreen(77)"=300, "SLODiffThreshBlue(78)"=300}  # ST SLO Threshold
      w173 = T20 {"disableSADColor(68)"=0, "disableRAUColor(69)"=0, "disableSLORightColor(70)"=0, "disableSLOLeftColor(71)"=0, "disableSADNormalize(72)"=0}  # ST Color Control
      w174 = T17 {"rauDiffThreshRed(73)"=600, "rauDiffThreshGreen(74)"=600, "rauDiffThreshBlue(75)"=600}  # ST Rau Threshold
      w175 = T18 {"sloK1Penalty (79)"=44, "sloK2Penalty (80)"=502, "sloK1PenaltyMod1(81)"=23, "sloK2PenaltyMod1(82)"=237, "sloK1PenaltyMod2(83)"=219, "sloK2PenaltyMod2(84)"=113}  # ST SLO Penalty
      w176 = T21 {"plusIncrement (47)"=10, "MinusDecrement (46)"=10, "deepSeaMedianThreshold (48)"=528, "scoreThreshA(49)"=10, "scoreThreshB (50)"=1023, "textureDifferenceThreshold (52)"=0, "textureCountThreshold (51)"=0, "deepSea2ndPeakThresh.(53)"=27, "deepSeaNeighborThresh.(54)"=20, "LRAgreeThreshold (55)"=70}  # depth control
      w177 = T16 {"minWest (60)"=1, "minEast (61)"=1, "minWEsum (62)"=1, "minNorth (63)"=1, "minSouth (64)"=1, "minNSSum(65)"=1, "uStrink (66)"=1, "vShrink (67)"=1}  # ST RAU vector
      w178 = T13 {"rsmBypass (56)"=0, "diffThresh (57)"=7.0, "sloRauDiffThresh(58)"=3.0, "removeThresh(59)"=33}  # ST RSM
    }
    frame "Face2" {
      w180 = cluster{"uDiameter":u32, "vDiameter":u32} {"uDiameter"=9, "vDiameter"=9}  # ST_CensusEnable
      w181 = T15 {"depthUnits, um"=1000, "depthClampMin"=0, "depthClampMax"=65535, "disparityMultiplier"=0, "disparityShift(0-127)"=0}  # Depth Table
      w179 = cluster{"meanIntensitySetpoint":u32} {"meanIntensitySetpoint"=800}  # ST_AE_Control
      w183 = T13 {"rsmBypass (56)"=0, "diffThresh (57)"=1.21875, "sloRauDiffThresh(58)"=0.28125, "removeThresh(59)"=83}  # ST RSM
      w184 = T16 {"minWest (60)"=3, "minEast (61)"=2, "minWEsum (62)"=7, "minNorth (63)"=1, "minSouth (64)"=3, "minNSSum(65)"=6, "uStrink (66)"=4, "vShrink (67)"=0}  # ST RAU vector
      w185 = T17 {"rauDiffThreshRed(73)"=18, "rauDiffThreshGreen(74)"=113, "rauDiffThreshBlue(75)"=586}  # ST Rau Threshold
      w186 = T21 {"plusIncrement (47)"=10, "MinusDecrement (46)"=10, "deepSeaMedianThreshold (48)"=528, "scoreThreshA(49)"=10, "scoreThreshB (50)"=1023, "textureDifferenceThreshold (52)"=0, "textureCountThreshold (51)"=0, "deepSea2ndPeakThresh.(53)"=27, "deepSeaNeighborThresh.(54)"=20, "LRAgreeThreshold (55)"=70}  # depth control
      w187 = T20 {"disableSADColor(68)"=0, "disableRAUColor(69)"=0, "disableSLORightColor(70)"=0, "disableSLOLeftColor(71)"=0, "disableSADNormalize(72)"=0}  # ST Color Control
      w188 = T19 {"SLOdiffThreshRed(76)"=279, "SLODiffThreshGreen(77)"=200, "SLODiffThreshBlue(78)"=8}  # ST SLO Threshold
      w189 = T18 {"sloK1Penalty (79)"=55, "sloK2Penalty (80)"=235, "sloK1PenaltyMod1(81)"=326, "sloK2PenaltyMod1(82)"=506, "sloK1PenaltyMod2(83)"=134, "sloK2PenaltyMod2(84)"=206}  # ST SLO Penalty
    }
    frame "Best Box" {
      w191 = cluster{"uDiameter":u32, "vDiameter":u32} {"uDiameter"=9, "vDiameter"=9}  # ST_CensusEnable
      w192 = T15 {"depthUnits, um"=1000, "depthClampMin"=0, "depthClampMax"=65535, "disparityMultiplier"=0, "disparityShift(0-127)"=0}  # Depth Table
      w190 = cluster{"meanIntensitySetpoint":u32} {"meanIntensitySetpoint"=400}  # ST_AE_Control
      w194 = T13 {"rsmBypass (56)"=0, "diffThresh (57)"=1.21875, "sloRauDiffThresh(58)"=0.28125, "removeThresh(59)"=83}  # ST RSM
      w195 = T16 {"minWest (60)"=3, "minEast (61)"=2, "minWEsum (62)"=7, "minNorth (63)"=1, "minSouth (64)"=3, "minNSSum(65)"=6, "uStrink (66)"=4, "vShrink (67)"=0}  # ST RAU vector
      w196 = T17 {"rauDiffThreshRed(73)"=18, "rauDiffThreshGreen(74)"=113, "rauDiffThreshBlue(75)"=586}  # ST Rau Threshold
      w197 = T21 {"plusIncrement (47)"=10, "MinusDecrement (46)"=10, "deepSeaMedianThreshold (48)"=528, "scoreThreshA(49)"=10, "scoreThreshB (50)"=1023, "textureDifferenceThreshold (52)"=0, "textureCountThreshold (51)"=0, "deepSea2ndPeakThresh.(53)"=27, "deepSeaNeighborThresh.(54)"=20, "LRAgreeThreshold (55)"=70}  # depth control
      w198 = T20 {"disableSADColor(68)"=0, "disableRAUColor(69)"=0, "disableSLORightColor(70)"=0, "disableSLOLeftColor(71)"=0, "disableSADNormalize(72)"=0}  # ST Color Control
      w199 = T19 {"SLOdiffThreshRed(76)"=279, "SLODiffThreshGreen(77)"=200, "SLODiffThreshBlue(78)"=8}  # ST SLO Threshold
      w200 = T18 {"sloK1Penalty (79)"=55, "sloK2Penalty (80)"=235, "sloK1PenaltyMod1(81)"=326, "sloK2PenaltyMod1(82)"=506, "sloK1PenaltyMod2(83)"=134, "sloK2PenaltyMod2(84)"=206}  # ST SLO Penalty
    }
    frame "High Density" {
      n2 = Unbundle By Name(T14 {"depth control"={"plusIncrement"=21, "MinusDecrement"=6, "deepSeaMedianThreshold"=789, "scoreThreshA"=96, "scoreThreshB"=1443, "textureDifferenceThreshold"=2466, "textureCountThreshold"=0, "deepSeaSecondPeakThreshold"=222, "deepSeaNeighborThreshold"=12, "IrAgreeThreshold"=18}, "STColorCorrection output"={"colorCorrection 1"=0.54785156, "colorCorrection 2"=0.32910156, "colorCorrection 3"=0.8222656, "colorCorrection 4"=0.109375, "colorCorrection 5"=-0.40527344, "colorCorrection 6"=-1.5253906, "colorCorrection 7"=0.95703125, "colorCorrection 8"=0.89160156, "colorCorrection 9"=0.7675781, "colorCorrection 10"=-0.4794922, "colorCorrection 11"=0.047851562, "colorCorrection 12"=-0.2705078}, "HDAD"={"lambdaCensus"=15.0, "lambdaAD"=618.0, "ignoreSAD"=0}, "ST RSM"={"rsmBypass"=0, "diffThresh"=1.21875, "sloRauDiffThresh"=0.28125, "removeThresh"=82}, "ST SLO Penalty"={"sloK1Penalty"=55, "sloK2Penalty"=235, "sloK1PenaltyMod1"=326, "sloK2PenaltyMod1"=506, "sloK1PenaltyMod2"=134, "sloK2PenaltyMod2"=206}, "ST SLO Threshold"={"SLOdiffThresholdRed"=279, "SLODiffThresholdGreen"=200, "SLODiffThresholdBlue"=8}, "ST Rau Threshold"={"rauDiffThresholdRed"=18, "rauDiffThresholdGreen"=585, "rauDiffThresholdBlue"=112}, "ST Color Control"={"disableSADColor"=0, "disableRAUColor"=0, "disableSLORightColor"=0, "disableSLOLeftColor"=0, "disableSADNormalize"=0}, "ST RAU vector"={"minWest"=3, "minEast"=2, "minWEsum"=7, "minNorth"=1, "minSouth"=3, "minNSSum"=6, "uStrink"=4, "vShrink"=0}, "Depth Table"={"depthUnits, um"=1000, "depthClampMin"=0, "depthClampMax"=65535, "disparityMultiplier"=0, "disparityShift"=0}, "ST_AE_Control"={"meanIntensitySetpoint"=800}, "ST_CensusEnable"={"uDiameter"=9, "vDiameter"=9}} ("depth settings 2")) -> ("depth control"=w204:T4, "HDAD"=w210:T12, "ST RSM"=w209:T10, "ST SLO Penalty"=w201:T5, "ST SLO Threshold"=w202:T6, "ST Rau Threshold"=w207:T7, "ST Color Control"=w203:T8, "ST RAU vector"=w211:T9, "Depth Table"=w208:T3, "ST_AE_Control"=w205:cluster{"meanIntensitySetpoint":u32}, "ST_CensusEnable"=w206:cluster{"uDiameter":u32, "vDiameter":u32})  [unwired: 1 out]
    }
    frame "Medium Density" {
      n3 = Unbundle By Name(T14 {"depth control"={"plusIncrement"=3, "MinusDecrement"=23, "deepSeaMedianThreshold"=1021, "scoreThreshA"=54, "scoreThreshB"=887, "textureDifferenceThreshold"=0, "textureCountThreshold"=0, "deepSeaSecondPeakThreshold"=600, "deepSeaNeighborThreshold"=97, "IrAgreeThreshold"=19}, "STColorCorrection output"={"colorCorrection 1"=0.4013672, "colorCorrection 2"=0.047851562, "colorCorrection 3"=1.9179688, "colorCorrection 4"=0.54785156, "colorCorrection 5"=-1.5996094, "colorCorrection 6"=-0.48339844, "colorCorrection 7"=1.3095703, "colorCorrection 8"=0.79003906, "colorCorrection 9"=1.9511719, "colorCorrection 10"=-1.9951172, "colorCorrection 11"=0.8769531, "colorCorrection 12"=-0.70410156}, "HDAD"={"lambdaCensus"=26.0, "lambdaAD"=935.0, "ignoreSAD"=0}, "ST RSM"={"rsmBypass"=0, "diffThresh"=1.8125, "sloRauDiffThresh"=1.0, "removeThresh"=81}, "ST SLO Penalty"={"sloK1Penalty"=132, "sloK2Penalty"=342, "sloK1PenaltyMod1"=77, "sloK2PenaltyMod1"=390, "sloK1PenaltyMod2"=234, "sloK2PenaltyMod2"=151}, "ST SLO Threshold"={"SLOdiffThresholdRed"=896, "SLODiffThresholdGreen"=259, "SLODiffThresholdBlue"=16}, "ST Rau Threshold"={"rauDiffThresholdRed"=186, "rauDiffThresholdGreen"=723, "rauDiffThresholdBlue"=14}, "ST Color Control"={"disableSADColor"=0, "disableRAUColor"=0, "disableSLORightColor"=1, "disableSLOLeftColor"=0, "disableSADNormalize"=0}, "ST RAU vector"={"minWest"=5, "minEast"=3, "minWEsum"=11, "minNorth"=1, "minSouth"=3, "minNSSum"=6, "uStrink"=3, "vShrink"=1}, "Depth Table"={"depthUnits, um"=1000, "depthClampMin"=0, "depthClampMax"=65535, "disparityMultiplier"=0, "disparityShift"=0}, "ST_AE_Control"={"meanIntensitySetpoint"=800}, "ST_CensusEnable"={"uDiameter"=9, "vDiameter"=9}} ("depth settings 2")) -> ("depth control"=w217:T4, "HDAD"=w223:T12, "ST RSM"=w222:T10, "ST SLO Penalty"=w214:T5, "ST SLO Threshold"=w215:T6, "ST Rau Threshold"=w220:T7, "ST Color Control"=w216:T8, "ST RAU vector"=w224:T9, "Depth Table"=w221:T3, "ST_AE_Control"=w218:cluster{"meanIntensitySetpoint":u32}, "ST_CensusEnable"=w219:cluster{"uDiameter":u32, "vDiameter":u32})  [unwired: 1 out]
    }
    frame "High Accuracy" {
      n4 = Unbundle By Name(T14 {"depth control"={"plusIncrement"=2, "MinusDecrement"=25, "deepSeaMedianThreshold"=796, "scoreThreshA"=4, "scoreThreshB"=2893, "textureDifferenceThreshold"=1722, "textureCountThreshold"=0, "deepSeaSecondPeakThreshold"=647, "deepSeaNeighborThreshold"=108, "IrAgreeThreshold"=10}, "STColorCorrection output"={"colorCorrection 1"=0.4013672, "colorCorrection 2"=0.047851562, "colorCorrection 3"=1.9179688, "colorCorrection 4"=0.54785156, "colorCorrection 5"=-1.5996094, "colorCorrection 6"=-0.48339844, "colorCorrection 7"=1.3095703, "colorCorrection 8"=0.79003906, "colorCorrection 9"=1.9511719, "colorCorrection 10"=-1.9951172, "colorCorrection 11"=0.8769531, "colorCorrection 12"=-0.70410156}, "HDAD"={"lambdaCensus"=26.0, "lambdaAD"=935.0, "ignoreSAD"=0}, "ST RSM"={"rsmBypass"=0, "diffThresh"=1.65625, "sloRauDiffThresh"=0.71875, "removeThresh"=137}, "ST SLO Penalty"={"sloK1Penalty"=155, "sloK2Penalty"=190, "sloK1PenaltyMod1"=160, "sloK2PenaltyMod1"=507, "sloK1PenaltyMod2"=59, "sloK2PenaltyMod2"=493}, "ST SLO Threshold"={"SLOdiffThresholdRed"=30, "SLODiffThresholdGreen"=15, "SLODiffThresholdBlue"=13}, "ST Rau Threshold"={"rauDiffThresholdRed"=1007, "rauDiffThresholdGreen"=578, "rauDiffThresholdBlue"=803}, "ST Color Control"={"disableSADColor"=0, "disableRAUColor"=0, "disableSLORightColor"=1, "disableSLOLeftColor"=0, "disableSADNormalize"=0}, "ST RAU vector"={"minWest"=2, "minEast"=6, "minWEsum"=12, "minNorth"=3, "minSouth"=2, "minNSSum"=7, "uStrink"=3, "vShrink"=0}, "Depth Table"={"depthUnits, um"=1000, "depthClampMin"=0, "depthClampMax"=65535, "disparityMultiplier"=0, "disparityShift"=0}, "ST_AE_Control"={"meanIntensitySetpoint"=800}, "ST_CensusEnable"={"uDiameter"=9, "vDiameter"=9}} ("depth settings 2")) -> ("depth control"=w229:T4, "HDAD"=w235:T12, "ST RSM"=w234:T10, "ST SLO Penalty"=w226:T5, "ST SLO Threshold"=w227:T6, "ST Rau Threshold"=w232:T7, "ST Color Control"=w228:T8, "ST RAU vector"=w236:T9, "Depth Table"=w233:T3, "ST_AE_Control"=w230:cluster{"meanIntensitySetpoint":u32}, "ST_CensusEnable"=w231:cluster{"uDiameter":u32, "vDiameter":u32})  [unwired: 1 out]
    }
    frame "Hand" {
      n5 = Unbundle By Name(T14 {"depth control"={"plusIncrement"=3, "MinusDecrement"=20, "deepSeaMedianThreshold"=240, "scoreThreshA"=24, "scoreThreshB"=791, "textureDifferenceThreshold"=783, "textureCountThreshold"=0, "deepSeaSecondPeakThreshold"=31, "deepSeaNeighborThreshold"=110, "IrAgreeThreshold"=20}, "STColorCorrection output"={"colorCorrection 1"=0.4013672, "colorCorrection 2"=0.047851562, "colorCorrection 3"=1.9179688, "colorCorrection 4"=0.54785156, "colorCorrection 5"=-1.5996094, "colorCorrection 6"=-0.48339844, "colorCorrection 7"=1.3095703, "colorCorrection 8"=0.79003906, "colorCorrection 9"=1.9511719, "colorCorrection 10"=-1.9951172, "colorCorrection 11"=0.8769531, "colorCorrection 12"=-0.70410156}, "HDAD"={"lambdaCensus"=7.0, "lambdaAD"=1001.0, "ignoreSAD"=0}, "ST RSM"={"rsmBypass"=0, "diffThresh"=3.8125, "sloRauDiffThresh"=0.46875, "removeThresh"=94}, "ST SLO Penalty"={"sloK1Penalty"=63, "sloK2Penalty"=45, "sloK1PenaltyMod1"=14, "sloK2PenaltyMod1"=21, "sloK1PenaltyMod2"=119, "sloK2PenaltyMod2"=12}, "ST SLO Threshold"={"SLOdiffThresholdRed"=618, "SLODiffThresholdGreen"=244, "SLODiffThresholdBlue"=130}, "ST Rau Threshold"={"rauDiffThresholdRed"=141, "rauDiffThresholdGreen"=74, "rauDiffThresholdBlue"=50}, "ST Color Control"={"disableSADColor"=0, "disableRAUColor"=0, "disableSLORightColor"=1, "disableSLOLeftColor"=0, "disableSADNormalize"=0}, "ST RAU vector"={"minWest"=1, "minEast"=3, "minWEsum"=14, "minNorth"=1, "minSouth"=3, "minNSSum"=4, "uStrink"=3, "vShrink"=1}, "Depth Table"={"depthUnits, um"=1000, "depthClampMin"=0, "depthClampMax"=65535, "disparityMultiplier"=0, "disparityShift"=0}, "ST_AE_Control"={"meanIntensitySetpoint"=800}, "ST_CensusEnable"={"uDiameter"=9, "vDiameter"=9}} ("depth settings 2")) -> ("depth control"=w241:T4, "HDAD"=w247:T12, "ST RSM"=w246:T10, "ST SLO Penalty"=w238:T5, "ST SLO Threshold"=w239:T6, "ST Rau Threshold"=w244:T7, "ST Color Control"=w240:T8, "ST RAU vector"=w248:T9, "Depth Table"=w245:T3, "ST_AE_Control"=w242:cluster{"meanIntensitySetpoint":u32}, "ST_CensusEnable"=w243:cluster{"uDiameter":u32, "vDiameter":u32})  [unwired: 1 out]
    }
    frame "Short Range" {
      n6 = Unbundle By Name(T14 {"depth control"={"plusIncrement"=10, "MinusDecrement"=10, "deepSeaMedianThreshold"=528, "scoreThreshA"=10, "scoreThreshB"=1023, "textureDifferenceThreshold"=0, "textureCountThreshold"=0, "deepSeaSecondPeakThreshold"=27, "deepSeaNeighborThreshold"=20, "IrAgreeThreshold"=70}, "STColorCorrection output"={"colorCorrection 1"=0.4013672, "colorCorrection 2"=0.047851562, "colorCorrection 3"=1.9179688, "colorCorrection 4"=0.54785156, "colorCorrection 5"=-1.5996094, "colorCorrection 6"=-0.48339844, "colorCorrection 7"=1.3095703, "colorCorrection 8"=0.79003906, "colorCorrection 9"=1.9511719, "colorCorrection 10"=-1.9951172, "colorCorrection 11"=0.8769531, "colorCorrection 12"=-0.70410156}, "HDAD"={"lambdaCensus"=26.0, "lambdaAD"=935.0, "ignoreSAD"=0}, "ST RSM"={"rsmBypass"=0, "diffThresh"=7.0, "sloRauDiffThresh"=3.0, "removeThresh"=32}, "ST SLO Penalty"={"sloK1Penalty"=44, "sloK2Penalty"=502, "sloK1PenaltyMod1"=23, "sloK2PenaltyMod1"=237, "sloK1PenaltyMod2"=219, "sloK2PenaltyMod2"=113}, "ST SLO Threshold"={"SLOdiffThresholdRed"=300, "SLODiffThresholdGreen"=300, "SLODiffThresholdBlue"=300}, "ST Rau Threshold"={"rauDiffThresholdRed"=599, "rauDiffThresholdGreen"=599, "rauDiffThresholdBlue"=599}, "ST Color Control"={"disableSADColor"=0, "disableRAUColor"=0, "disableSLORightColor"=0, "disableSLOLeftColor"=0, "disableSADNormalize"=0}, "ST RAU vector"={"minWest"=1, "minEast"=1, "minWEsum"=1, "minNorth"=1, "minSouth"=1, "minNSSum"=1, "uStrink"=1, "vShrink"=1}, "Depth Table"={"depthUnits, um"=1000, "depthClampMin"=0, "depthClampMax"=65535, "disparityMultiplier"=0, "disparityShift"=0}, "ST_AE_Control"={"meanIntensitySetpoint"=800}, "ST_CensusEnable"={"uDiameter"=9, "vDiameter"=9}} ("depth settings 2")) -> ("depth control"=w253:T4, "HDAD"=w259:T12, "ST RSM"=w258:T10, "ST SLO Penalty"=w250:T5, "ST SLO Threshold"=w251:T6, "ST Rau Threshold"=w256:T7, "ST Color Control"=w252:T8, "ST RAU vector"=w260:T9, "Depth Table"=w257:T3, "ST_AE_Control"=w254:cluster{"meanIntensitySetpoint":u32}, "ST_CensusEnable"=w255:cluster{"uDiameter":u32, "vDiameter":u32})  [unwired: 1 out]
    }
    frame "Flat wall" {
      # "AndersDepth4"
      n7 = Unbundle By Name(T14 {"depth control"={"plusIncrement"=10, "MinusDecrement"=10, "deepSeaMedianThreshold"=528, "scoreThreshA"=10, "scoreThreshB"=1023, "textureDifferenceThreshold"=0, "textureCountThreshold"=0, "deepSeaSecondPeakThreshold"=27, "deepSeaNeighborThreshold"=20, "IrAgreeThreshold"=70}, "STColorCorrection output"={"colorCorrection 1"=0.4013672, "colorCorrection 2"=0.047851562, "colorCorrection 3"=1.9179688, "colorCorrection 4"=0.54785156, "colorCorrection 5"=-1.5996094, "colorCorrection 6"=-0.48339844, "colorCorrection 7"=1.3095703, "colorCorrection 8"=0.79003906, "colorCorrection 9"=1.9511719, "colorCorrection 10"=-1.9951172, "colorCorrection 11"=0.8769531, "colorCorrection 12"=-0.70410156}, "HDAD"={"lambdaCensus"=26.0, "lambdaAD"=935.0, "ignoreSAD"=0}, "ST RSM"={"rsmBypass"=0, "diffThresh"=7.0, "sloRauDiffThresh"=3.0, "removeThresh"=32}, "ST SLO Penalty"={"sloK1Penalty"=44, "sloK2Penalty"=502, "sloK1PenaltyMod1"=23, "sloK2PenaltyMod1"=237, "sloK1PenaltyMod2"=219, "sloK2PenaltyMod2"=113}, "ST SLO Threshold"={"SLOdiffThresholdRed"=300, "SLODiffThresholdGreen"=300, "SLODiffThresholdBlue"=300}, "ST Rau Threshold"={"rauDiffThresholdRed"=599, "rauDiffThresholdGreen"=599, "rauDiffThresholdBlue"=599}, "ST Color Control"={"disableSADColor"=0, "disableRAUColor"=0, "disableSLORightColor"=0, "disableSLOLeftColor"=0, "disableSADNormalize"=0}, "ST RAU vector"={"minWest"=1, "minEast"=1, "minWEsum"=1, "minNorth"=1, "minSouth"=1, "minNSSum"=1, "uStrink"=1, "vShrink"=1}, "Depth Table"={"depthUnits, um"=1000, "depthClampMin"=0, "depthClampMax"=65535, "disparityMultiplier"=0, "disparityShift"=0}, "ST_AE_Control"={"meanIntensitySetpoint"=800}, "ST_CensusEnable"={"uDiameter"=9, "vDiameter"=9}} ("depth settings 2")) -> ("depth control"=w265:T4, "HDAD"=w271:T12, "ST RSM"=w270:T10, "ST SLO Penalty"=w262:T5, "ST SLO Threshold"=w263:T6, "ST Rau Threshold"=w268:T7, "ST Color Control"=w264:T8, "ST RAU vector"=w272:T9, "Depth Table"=w269:T3, "ST_AE_Control"=w266:cluster{"meanIntensitySetpoint":u32}, "ST_CensusEnable"=w267:cluster{"uDiameter":u32, "vDiameter":u32})  [unwired: 1 out]
    }
    frame "Load .JSON" {
      w274 = cluster{"uDiameter":u32, "vDiameter":u32} {"uDiameter"=9, "vDiameter"=9}  # ST_CensusEnable
      w275 = T15 {"depthUnits, um"=1000, "depthClampMin"=0, "depthClampMax"=65535, "disparityMultiplier"=0, "disparityShift(0-127)"=0}  # Depth Table
      w273 = cluster{"meanIntensitySetpoint":u32} {"meanIntensitySetpoint"=400}  # ST_AE_Control
      n8 = call "File Dialog"("prompt"="Load .JSON file", "pattern (all files)"="*.json") -> ("selected path"=w278:path)  [unwired: 10 in, 3 out]
      n9 = call <vilib>:"rs3_ReadDepthPreference3.vi"("file (use dialog)"=w278) -> ("HDAD 2*"=w281:T12, "ST Color Control 2"=w286:T20, "depth control 2"=w280:T22, "ST RSM 2"=w282:T13, "ST SLO Penalty 2"=w284:T18, "ST SLO Threshold 2"=w285:T19, "ST Rau Threshold 2"=w283:T17, "ST RAU vector 2"=w279:T16)  [unwired: 5 in, 2 out]
    }
    frame "Load .JSON2" {
      n10 = call "File Dialog2"("prompt"="Load .JSON file", "pattern (all files)"="*.json") -> ("selected path"=w292:path)  [unwired: 10 in, 3 out]
      n11 = call <vilib>:"rs3_ReadDepthPreference4.vi"("file (use dialog)"=w292) -> ("HDAD 2*"=w295:T12, "ST_AE_Control"=w289:cluster{"meanIntensitySetpoint":u32}, "ST Color Control 2"=w300:T20, "depth control 2"=w294:T22, "ST RSM 2"=w296:T13, "Depth Table"=w287:T15, "ST SLO Penalty 2"=w298:T18, "ST_CensusEnable"=w288:cluster{"uDiameter":u32, "vDiameter":u32}, "ST SLO Threshold 2"=w299:T19, "ST Rau Threshold 2"=w297:T17, "ST RAU vector 2"=w293:T16)  [unwired: 2 in, 2 out]
    }
  }
  n12 = case shown="\"RS400 (DS5p)\", Default" "Color Presets" {
    tunnel: [w301 T23 {"DS5p- 1"=0.30136988, "colorCorrection 2"=-0.05479452, "colorCorrection 3"=1.9726027, "colorCorrection 4"=0.9041096, "colorCorrection 5"=-0.41095892, "colorCorrection 6"=-1.6438357, "colorCorrection 7"=0.63013697, "colorCorrection 8"=1.7534246, "colorCorrection 9"=1.5068493, "colorCorrection 10"=-2.0, "colorCorrection 11"=1.9726027, "colorCorrection 12"=-1.2876712} ("STColorCorrection") T11 {"colorCorrection 1"=1.339452, "colorCorrection 2"=0.045342464, "colorCorrection 3"=0.80136985, "colorCorrection 4"=0.19479452, "colorCorrection 5"=-1.2150685, "colorCorrection 6"=-0.9254795, "colorCorrection 7"=0.4671233, "colorCorrection 8"=1.3315068, "colorCorrection 9"=1.7899219, "colorCorrection 10"=-1.1794521, "colorCorrection 11"=0.0779452, "colorCorrection 12"=0.049178082} ("STColorCorrection") T11 {"colorCorrection 1"=0.21917808, "colorCorrection 2"=-0.1369863, "colorCorrection 3"=0.79452056, "colorCorrection 4"=0.69452053, "colorCorrection 5"=-0.28095892, "colorCorrection 6"=-1.7138357, "colorCorrection 7"=0.78013694, "colorCorrection 8"=1.4534247, "colorCorrection 9"=0.9368493, "colorCorrection 10"=-1.7, "colorCorrection 11"=1.6836027, "colorCorrection 12"=-0.8076712} ("STColorCorrection") T11 {"colorCorrection 1"=0.5479452, "colorCorrection 2"=0.32876712, "colorCorrection 3"=0.82191783, "colorCorrection 4"=0.10958904, "colorCorrection 5"=-0.4050685, "colorCorrection 6"=-1.5254794, "colorCorrection 7"=0.9571233, "colorCorrection 8"=0.89150685, "colorCorrection 9"=1.189922, "colorCorrection 10"=-0.47945204, "colorCorrection 11"=0.047945205, "colorCorrection 12"=-0.27082193} ("STColorCorrection") T11 {"colorCorrection 1"=0.5479452, "colorCorrection 2"=0.32876712, "colorCorrection 3"=0.37, "colorCorrection 4"=0.11958904, "colorCorrection 5"=-0.044, "colorCorrection 6"=-1.43, "colorCorrection 7"=0.707, "colorCorrection 8"=0.89050686, "colorCorrection 9"=0.766922, "colorCorrection 10"=-0.47945204, "colorCorrection 11"=0.2099452, "colorCorrection 12"=-0.28982192} ("STColorCorrection") w307 T11 {"colorCorrection 1"=-0.1369863, "colorCorrection 2"=1.3424658, "colorCorrection 3"=1.6986301, "colorCorrection 4"=1.7534246, "colorCorrection 5"=-0.8767123, "colorCorrection 6"=-1.9452055, "colorCorrection 7"=1.4520547, "colorCorrection 8"=1.5616438, "colorCorrection 9"=1.479452, "colorCorrection 10"=-2.0, "colorCorrection 11"=1.3972603, "colorCorrection 12"=-0.65753424} ("STColorCorrection") T11 {"colorCorrection 1"=0.30136988, "colorCorrection 2"=-0.05479452, "colorCorrection 3"=1.9726027, "colorCorrection 4"=0.9041096, "colorCorrection 5"=-0.7123288, "colorCorrection 6"=-2.0, "colorCorrection 7"=0.79452056, "colorCorrection 8"=1.99, "colorCorrection 9"=1.3468493, "colorCorrection 10"=-2.0, "colorCorrection 11"=1.8466027, "colorCorrection 12"=-1.3068492} ("STColorCorrection") T11 {"colorCorrection 1"=0.5479452, "colorCorrection 2"=0.32876712, "colorCorrection 3"=0.82191783, "colorCorrection 4"=0.10958904, "colorCorrection 5"=-0.4050685, "colorCorrection 6"=-1.5254794, "colorCorrection 7"=0.9571233, "colorCorrection 8"=0.89150685, "colorCorrection 9"=0.7671233, "colorCorrection 10"=-0.47945204, "colorCorrection 11"=0.047945205, "colorCorrection 12"=-0.27082193} ("STColorCorrection") T11 {"colorCorrection 1"=0.40136987, "colorCorrection 2"=0.047945205, "colorCorrection 3"=1.9178082, "colorCorrection 4"=0.5479452, "colorCorrection 5"=-1.5999494, "colorCorrection 6"=-0.48342466, "colorCorrection 7"=1.3093151, "colorCorrection 8"=0.79, "colorCorrection 9"=1.9508219, "colorCorrection 10"=-1.9952055, "colorCorrection 11"=0.87660265, "colorCorrection 12"=-0.7039726} ("STColorCorrection") w312 w313 w314 w315 w316 T11 {"colorCorrection 1"=0.5479452, "colorCorrection 2"=1.3701172, "colorCorrection 3"=0.65722656, "colorCorrection 4"=0.60253906, "colorCorrection 5"=1.99, "colorCorrection 6"=0.19178082, "colorCorrection 7"=-1.2602739, "colorCorrection 8"=-0.5751953, "colorCorrection 9"=-0.43835616, "colorCorrection 10"=0.24609375, "colorCorrection 11"=-0.7675781, "colorCorrection 12"=1.3154297} ("STColorCorrection") T11 {"colorCorrection 1"=0.12988281, "colorCorrection 2"=0.39941406, "colorCorrection 3"=0.39941406, "colorCorrection 4"=-0.06933594, "colorCorrection 5"=-0.19824219, "colorCorrection 6"=-0.4033203, "colorCorrection 7"=-0.4033203, "colorCorrection 8"=1.0058594, "colorCorrection 9"=0.921875, "colorCorrection 10"=-0.44140625, "colorCorrection 11"=-0.44140625, "colorCorrection 12"=-0.0390625} ("Read color")] -> w2
    tunnel: "STColorCorrection" -> [w301 _ _ _ _ _ _ _ _ _ _ _ _ _ _ _ _ _]
    frame "Custom" {
    }
    frame "RS400 (DS5p)", Default {
    }
    frame "RS400 (DS5p) 2" {
    }
    frame "RS400 (DS5p) 3" {
    }
    frame "RS400 (DS5p) 4" {
    }
    frame "RS400 (DS5p) 5" {
    }
    frame "RS410 (DS5a)" {
      w307 = T11 {"colorCorrection 1"=0.30136988, "colorCorrection 2"=-0.05479452, "colorCorrection 3"=1.9726027, "colorCorrection 4"=0.9041096, "colorCorrection 5"=-0.84931505, "colorCorrection 6"=-1.8082192, "colorCorrection 7"=1.3424658, "colorCorrection 8"=1.7808219, "colorCorrection 9"=1.5068493, "colorCorrection 10"=-2.0, "colorCorrection 11"=1.9726027, "colorCorrection 12"=-1.2876712}  # DS5p
    }
    frame "RS410 (DS5a) 2" {
    }
    frame "DS410 (DS5a) 3" {
    }
    frame "DS410 (DS5a) 4" {
    }
    frame "DS410+IR" {
    }
    frame "DS5LR" {
      w312 = T24 {"Color 0"=0.795, "Color 1"=0.71, "Color 2"=0.493, "Color 3"=0.11, "Color 4"=-0.329, "Color 5"=-1.5902739726027402, "Color 6"=1.1, "Color 7"=1.04, "Color 8"=1.01, "Color 9"=-0.479, "Color 10"=-0.164, "Color 11"=-0.274}  # DS5LR
    }
    frame "DS5LR-2" {
      w313 = T24 {"Color 0"=0.2988, "Color 1"=0.2939, "Color 2"=0.2939, "Color 3"=0.114, "Color 4"=-0.1689, "Color 5"=-0.0849, "Color 6"=-0.0849, "Color 7"=0.5, "Color 8"=0.5, "Color 9"=-0.148, "Color 10"=-0.2109, "Color 11"=-0.081}  # DS5LR1
    }
    frame "DS5LR no pattern" {
      w314 = T24 {"Color 0"=1.9178082191780819, "Color 1"=1.99, "Color 2"=-2.0, "Color 3"=-2.0, "Color 4"=-1.041095890410959, "Color 5"=0.05479452054794498, "Color 6"=-0.2191780821917808, "Color 7"=0.904109589041096, "Color 8"=0.904109589041096, "Color 9"=-0.547945205479452, "Color 10"=-0.13698630136986312, "Color 11"=-0.19178082191780832}  # DS5LR no IR pattern
    }
    frame "RS410 Remove IR" {
      w315 = T24 {"Color 0"=0.4384765625, "Color 1"=1.990234375, "Color 2"=1.990234375, "Color 3"=-2.0, "Color 4"=-1.83984375, "Color 5"=-0.21875, "Color 6"=1.009765625, "Color 7"=1.33984375, "Color 8"=1.73046875, "Color 9"=-1.9951171875, "Color 10"=0.5751953125, "Color 11"=-0.4931640625}  # DS5 no pattern
    }
    frame "RS410 Remove IR 2" {
      w316 = T24 {"Color 0"=0.5205479452054793, "Color 1"=1.99, "Color 2"=1.506849315068493, "Color 3"=-2.0, "Color 4"=-2.0, "Color 5"=-0.08219178082191791, "Color 6"=1.1232876712328768, "Color 7"=1.013698630136986, "Color 8"=1.698630136986301, "Color 9"=-2.0, "Color 10"=0.5753424657534243, "Color 11"=-0.41095890410958913}  # No pattern 3
    }
    frame "DS5micro" {
      (unwired) T11 {"colorCorrection 1"=1.3424658, "colorCorrection 2"=1.369863, "colorCorrection 3"=0.65753424, "colorCorrection 4"=0.60273975, "colorCorrection 5"=1.2876712, "colorCorrection 6"=-0.10958904, "colorCorrection 7"=-0.5753425, "colorCorrection 8"=-0.5753425, "colorCorrection 9"=-1.0410959, "colorCorrection 10"=0.24657534, "colorCorrection 11"=-0.7671233, "colorCorrection 12"=1.3150685} ("STColorCorrection 2")
      (unwired) T11 {"colorCorrection 1"=1.150685, "colorCorrection 2"=1.5068493, "colorCorrection 3"=1.6164384, "colorCorrection 4"=0.08219178, "colorCorrection 5"=1.99, "colorCorrection 6"=-0.7671233, "colorCorrection 7"=-0.82191783, "colorCorrection 8"=-0.60273975, "colorCorrection 9"=0.10958904, "colorCorrection 10"=0.19178082, "colorCorrection 11"=-1.369863, "colorCorrection 12"=1.9452055} ("STColorCorrection")
    }
    frame "D435" {
    }
  }
  n13 = call <vilib>:"rs3 Advanced Set Census Enable Reg3.vi"("error in (no error)"="error in (no error)", "ST_CensusEnableReg"=w8, "device in"="device in") -> ("error out 2"=w77:errorcluster, "error"=w45:u64, "Dev out"=w76:u64)  [unwired: 6 in]
  n14 = call <vilib>:"rs3 Advanced AE setpoint3.vi"("error in (no error)"=w77, "ST_AE_Control"=w6, "device in"=w76) -> ("error out"=w75:errorcluster, "error"=w43:u64, "Dev out"=w74:u64)  [unwired: 6 in]
  n15 = call <vilib>:"rs3 Advanced set depth table control3.vi"("error in (no error)"=w75, "Depth Table"=w4, "device in"=w74) -> ("error out 2"=w73:errorcluster, "error"=w41:u64, "Dev out"=w72:u64)  [unwired: 6 in]
  n16 = call <vilib>:"rs3 Advanced set depth control3.vi"("error in (no error)"=w73, "depth control"=w50, "device in"=w72) -> ("error out"=w71:errorcluster, "error"=w39:u64, "Dev out"=w70:u64)  [unwired: 6 in]
  n17 = call <vilib>:"rs3 Advanced set HDAD3.vi"("error in (no error)"=w71, "HDAD"=w48, "device in"=w70) -> ("error out"=w69:errorcluster, "error"=w38:u64, "Dev out"=w68:u64)  [unwired: 6 in]
  n18 = call <vilib>:"rs3 Advanced set SLO Penalty3.vi"("error in (no error)"=w69, "ST SLO Penalty"=w20, "device in"=w68) -> ("error out"=w67:errorcluster, "error"=w37:u64, "Dev out"=w66:u64)  [unwired: 6 in]
  n19 = call <vilib>:"rs3 Advanced set SLO Threshold3.vi"("error in (no error)"=w67, "ST SLO Threshold"=w17, "device in"=w66) -> ("error out"=w65:errorcluster, "error"=w36:u64, "Dev out"=w64:u64)  [unwired: 6 in]
  n20 = call <vilib>:"rs3 Advanced set RAU control3.vi"("error in (no error)"=w65, "ST RAU vector"=w14, "device in"=w64) -> ("error out"=w63:errorcluster, "error"=w35:u64, "Dev out"=w62:u64)  [unwired: 6 in]
  n21 = call <vilib>:"rs3 Advanced set Rau Threshold3.vi"("error in (no error)"=w63, "ST Rau Threshold"=w15, "device in"=w62) -> ("error out"=w61:errorcluster, "error"=w34:u64, "Dev out"=w60:u64)  [unwired: 6 in]
  n22 = case shown="True" "Set Color Corr" {
    tunnel: w61 -> [w320 w327]
    tunnel: w60 -> [w321 w326]
    tunnel: w2 -> [_ w325]
    tunnel: [w320 w324] -> w59
    tunnel: [w321 w323] -> w58
    tunnel: [u64 0 ("error") w322] -> w32
    frame False {
    }
    frame True {
      n23 = call <vilib>:"rs3 Advanced set color correction3.vi"("error in (no error)"=w327, "STColorCorrection input"=w325, "device in"=w326) -> ("error out"=w324:errorcluster, "error"=w322:u64, "Dev out"=w323:u64)  [unwired: 6 in]
    }
  }
  n24 = call <vilib>:"rs3 Advanced set Color control3.vi"("error in (no error)"=w59, "ST Color Control"=w10, "device in"=w58) -> ("error out"=w57:errorcluster, "error"=w31:u64, "Dev out"=w56:u64)  [unwired: 6 in]
  n25 = call <vilib>:"rs3 Advanced set RSM control3.vi"("error in (no error)"=w57, "ST RSM"=w12, "device in"=w56) -> ("error out"=→"error out":errorcluster, "error"=w33:u64, "Dev out"=→"Dev out":u64)  [unwired: 6 in]
  n26 = call <vilib>:"rs3 showError.vi"("error"=w45) -> ("Error summary"=w44:string)  [unwired: 6 in, 4 out]
  n27 = call <vilib>:"rs3 showError.vi"("error"=w43) -> ("Error summary"=w42:string)  [unwired: 6 in, 4 out]
  n28 = call <vilib>:"rs3 showError.vi"("error"=w41) -> ("Error summary"=w40:string)  [unwired: 6 in, 4 out]
  n29 = call <vilib>:"rs3 showError.vi"("error"=w39) -> ("Error summary"=w30:string)  [unwired: 6 in, 4 out]
  n30 = call <vilib>:"rs3 showError.vi"("error"=w38) -> ("Error summary"=w29:string)  [unwired: 6 in, 4 out]
  n31 = call <vilib>:"rs3 showError.vi"("error"=w37) -> ("Error summary"=w28:string)  [unwired: 6 in, 4 out]
  n32 = call <vilib>:"rs3 showError.vi"("error"=w36) -> ("Error summary"=w27:string)  [unwired: 6 in, 4 out]
  n33 = call <vilib>:"rs3 showError.vi"("error"=w35) -> ("Error summary"=w26:string)  [unwired: 6 in, 4 out]
  n34 = call <vilib>:"rs3 showError.vi"("error"=w33) -> ("Error summary"=w47:string)  [unwired: 6 in, 4 out]
  n35 = call <vilib>:"rs3 showError.vi"("error"=w34) -> ("Error summary"=w25:string)  [unwired: 6 in, 4 out]
  n36 = call <vilib>:"rs3 showError.vi"("error"=w32) -> ("Error summary"=w24:string)  [unwired: 6 in, 4 out]
  n37 = call <vilib>:"rs3 showError.vi"("error"=w31) -> ("Error summary"=w22:string)  [unwired: 6 in, 4 out]
  n38 = Concatenate Strings(w44, w23, w42, w23, w40, w23, w30, w23, w29, w23, w28, w23, w27, w23, w26, w23, w47, w23, w25, w23, w24, w23, w22) -> (→"Set advanced error":string)
